vi "takeoffland1.vi"() -> ()   [LabVIEW 2016]
uses:
  <vilib>/LVH/AR Drone Toolkit/Type Defs/AR Drone Resource.ctl
  <vilib>/LVH/AR Drone Toolkit/Decode NavData/Typedefs/NavData Demo.ctl
  <vilib>/LVH/AR Drone Toolkit/AR Drone.lvlib
panel:
  out "Video Stream":picture
  out "NavData Out":T1
  out "AR Drone Resource Out":T2={"UDP Control Connection"=refnum, "UDP NavData Connection"=refnum, "UDP Video Connection (Drone 1.0)"=refnum, "TCP Video Connection (Drone 2.0)"=refnum, "TCP Control Port Connection"=refnum, "Drone IP address"="192.168.1.1", "Drone Command Port"=5555, "Drone NavData Port"=5555, "Drone Vid Stream Port"=56828, "Drone TCP Control Port"=5559, "Home IP address"="192.168.1.2", "Home Command Port"=56828, "Home NavData Port"=56829, "Home Vid Stream Port"=56830, "Drone Version"=0, "Drone Index"=0, "Command Sequence"=0}
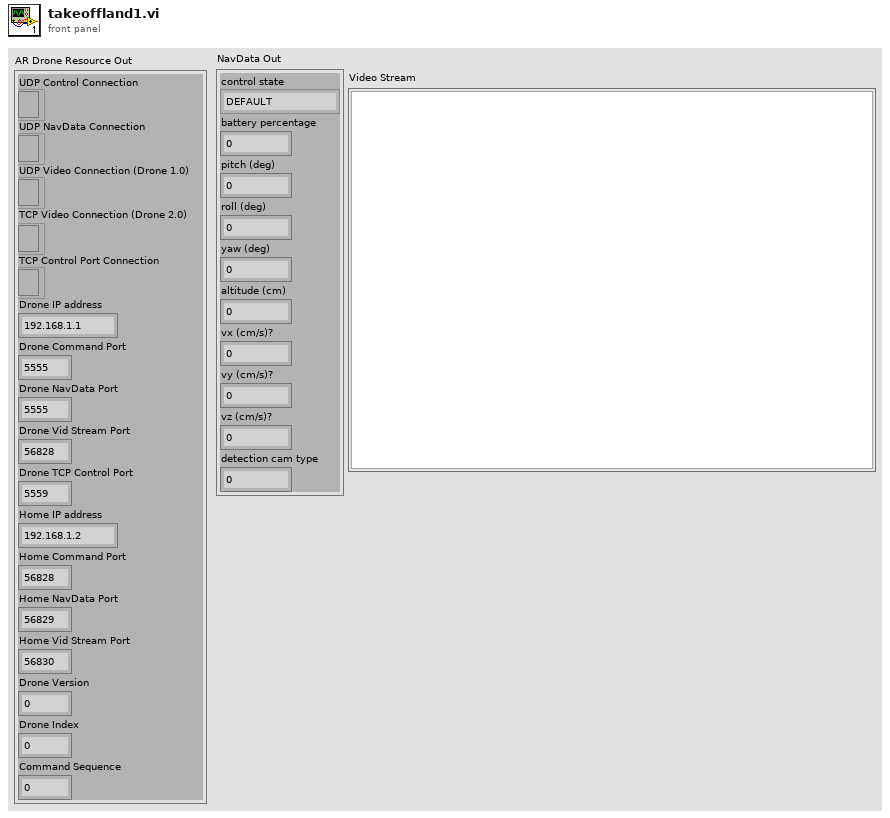
[diagram p1: front panel]
types:
  T1 = typedef "AR Drone.lvlib/NavData Demo.ctl" = cluster{"control state":enum32{"DEFAULT", "INIT", "LANDING", "FLYING", "HOVERING", "TEST", "TRANS_TAKEOFF", "TRANS_GOTOFIX", "TRANS_LANDING"}, "battery percentage":u32, "pitch (deg)":sgl, "roll (deg)":sgl, "yaw (deg)":sgl, "altitude (cm)":u32, "vx (cm/s)?":sgl, "vy (cm/s)?":sgl, "vz (cm/s)?":sgl, "detection cam type":u32}
  T2 = typedef "AR Drone.lvlib/AR Drone Resource.ctl" = cluster{"UDP Control Connection":refnum<k16>, "UDP NavData Connection":refnum<k16>, "UDP Video Connection (Drone 1.0)":refnum<k16>, "TCP Video Connection (Drone 2.0)":refnum<k5>, "TCP Control Port Connection":refnum<k5>, "Drone IP address":string, "Drone Command Port":u16, "Drone NavData Port":u16, "Drone Vid Stream Port":u16, "Drone TCP Control Port":u16, "Home IP address":string, "Home Command Port":u16, "Home NavData Port":u16, "Home Vid Stream Port":u16, "Drone Version":i32, "Drone Index":i32, "Command Sequence":i32}
  T3 = cluster{"Drone IP address":string, "Home IP address":string, "Flight Mode":enum8{"OUTDOOR MODE", "INDOOR MODE"}, "Mounted Hull":enum8{"OUTDOOR HULL", "INDOOR HULL"}, "Video Camera":u8, "Max Altitude (m)":sgl, "Max Pitch and Roll Angle (deg)":sgl, "Max Vertical Speed (m/s)":sgl, "Max Yaw Speed (deg/s)":sgl}
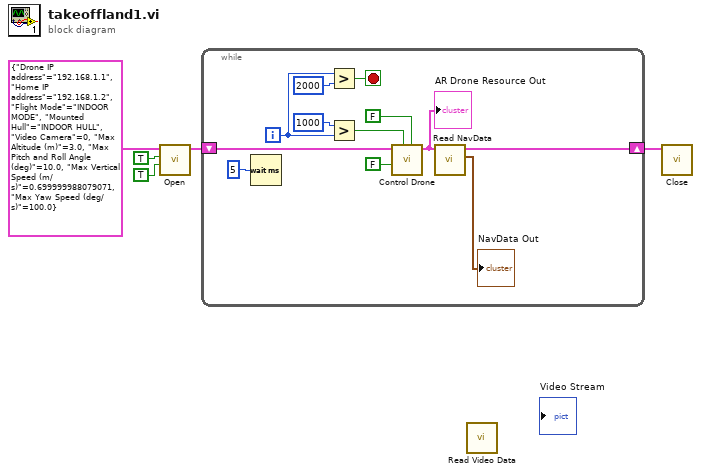
[diagram p0: block diagram]
diagram:
  n1 = call <vilib>:"Open.vi"("Init Video?"=TRUE, "Init NavData?"=TRUE, "Setup Parameters"=T3 {"Drone IP address"="192.168.1.1", "Home IP address"="192.168.1.2", "Flight Mode"=enum."INDOOR MODE", "Mounted Hull"=enum."INDOOR HULL", "Video Camera"=0, "Max Altitude (m)"=3.0, "Max Pitch and Roll Angle (deg)"=10.0, "Max Vertical Speed (m/s)"=0.7, "Max Yaw Speed (deg/s)"=100.0}) -> ("AR Drone Resource"=w2:T2)  [unwired: 7 in, 1 out]
  n2 = while {
    shift-right: [w6] -> w1
    shift-left: w2 -> [w17]
    i -> [w11]
    stop <- w9 stop-if-true
    n3 = Wait (ms)(milliseconds to wait=u32 5) -> ()  [unwired: 1 out]
    n4 = Greater?(x=w11, y=2000) -> (0:w9:bool)
    n5 = Greater?(x=1000 ("y"), y=w11) -> (0:w13:bool)
    n6 = call <vilib>:"Control Drone.vi"("Emergency Landing"=FALSE, "Takeoff/Land"=w13, "Hover"=FALSE, "AR Drone Resource"=w17) -> ("AR Drone Resource Out"=w8:T2)  [unwired: 6 in, 1 out]
    "AR Drone Resource Out" <- w8
    n7 = call <vilib>:"Read NavData.vi"("AR Drone Resource"=w8) -> ("NavData Out"=→"NavData Out":T1, "AR Drone Resource Out"=w6:T2)  [unwired: 8 in, 1 out]
  }
  n8 = call <vilib>:"Read Video Data.vi"() -> ()  [unwired: 9 in, 3 out]
  n9 = call <vilib>:"Close.vi"("AR Drone Resource"=w1) -> ()  [unwired: 10 in, 1 out]
